vi "LogSummary.vi"(8 "error in (no error)":errorcluster, 9 "Run Ratios":T1 {"LEC13/12" format="%_4e"; "DTfrac" format="%#_3g"; "DT" format="%#_3g"; "CountErr" format="%#_3g"; "d13C" format="%_4g"; "C13/12" format="%_4e"; "C14/12" format="%_4e"; "C14/13" format="%_3e"; "C12Cor" format="%_3e"; "C13" format="%_3e"; "C13H/L" format="%#_3g"}, 10 "Run Summary":T2 {"C12LE" format="%_3e"; "C13LE" format="%_3e"; "C1312" format="%_3e"; "C12" format="%_3e"; "C13L" format="%_3e"; "C13H" format="%_3e"}, 11 "Log File Path":path) -> (0 "error out":errorcluster)   [LabVIEW 2013]
uses:
  SummaryData.ctl
  RunRatios.ctl
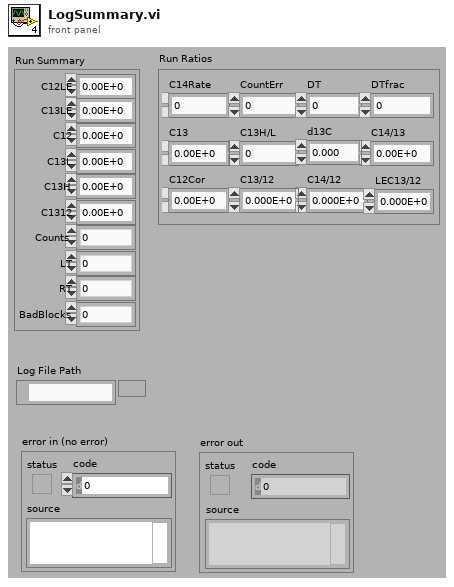
[diagram p1: front panel]
types:
  T1 = typedef "RunRatios.ctl" = cluster{"C14Rate":dbl, "CountErr":dbl, "DT":dbl, "DTfrac":dbl, "C13":dbl, "C13H/L":dbl, "d13C":dbl, "C14/13":dbl, "C12Cor":dbl, "C13/12":dbl, "C14/12":dbl, "LEC13/12":dbl}
  T2 = typedef "SummaryData.ctl" = cluster{"C12LE":dbl, "C13LE":dbl, "C12":dbl, "C13L":dbl, "C13H":dbl, "C1312":dbl, "Counts":u32, "LT":dbl, "RT":dbl, "BadBlocks":u8}
  T3 = enum16{"open", "replace", "create", "open or create", "replace or create", "replace or create with confirmation"}
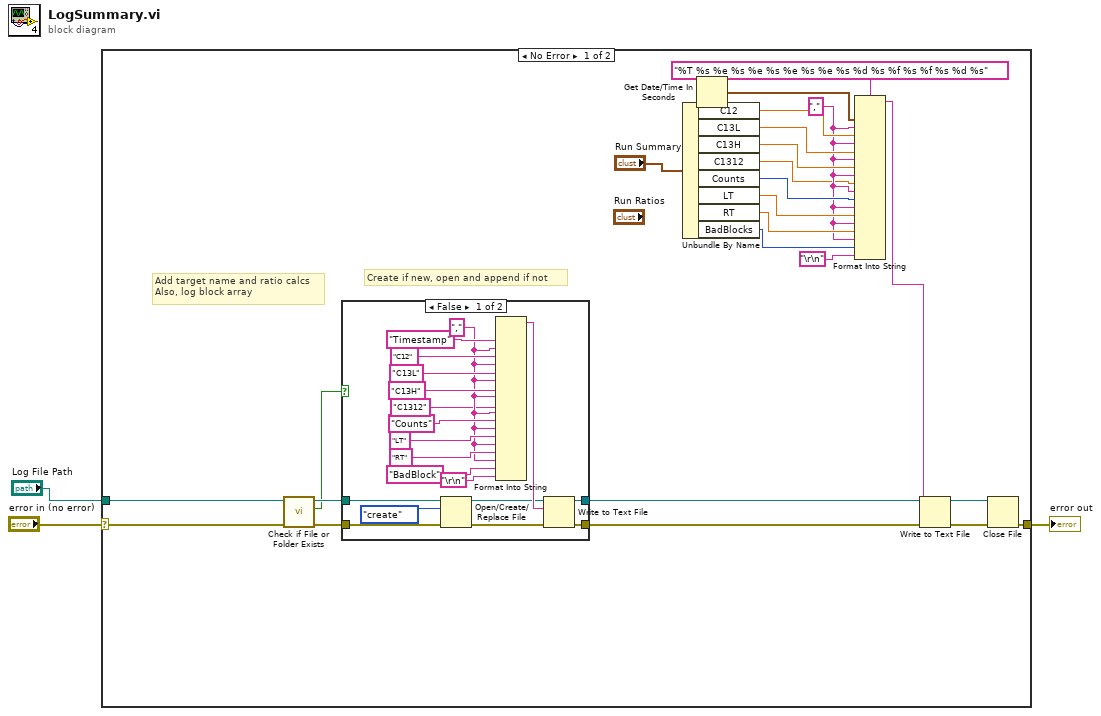
[diagram p0: block diagram]
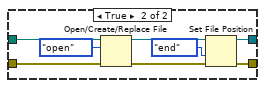
[diagram p2: hidden frame]
diagram:
  n1 = case shown="No Error" "error in (no error)" {
    selector: "error in (no error)" -> [w8 w55]
    tunnel: [w9 w55] -> w2
    tunnel: "Log File Path" -> [w4 _]
    frame No Error {
      w7 = ","
      # "Add target name and ratio calcs\nAlso, log block array"
      # "Create if new, open and append if not"
      n2 = call <vilib>:"Check if File or Folder Exists.vi"("error in (no error)"=w8, "path"=w4) -> ("error out"=w12:errorcluster, "file or folder exists?"=w10:bool, "dup path"=w13:path)  [unwired: 7 out]
      n3 = case shown="False" w10 {
        tunnel: [w33 w52] -> w16
        tunnel: [w32 w53] -> w11
        tunnel: w13 -> [w31 w49]
        tunnel: w12 -> [w30 w50]
        frame False {
          w29 = ","
          n4 = Open/Create/Replace File(file path (use dialog)=w31, error in=w30, operation (0:open)=T3."create") -> (refnum out=w35:refnum<file>, error out=w36:errorcluster)  [unwired: 4 out]
          n5 = Format Into String("Timestamp" ("input 1"), w29, "C12", w29, "C13L", w29, "C13H", w29, "C1312", w29, "Counts", w29, "LT", w29, "RT", w29, "BadBlock", "\r\n") -> (resulting string=w37:string)  [unwired: 3 in, 1 out]
          n6 = Write to Text File(file (use dialog)=w35, text=w37, error in=w36) -> (refnum out=w32:refnum<file>, error out=w33:errorcluster)  [unwired: 2 out]
        }
        frame True {
          n7 = Open/Create/Replace File(file path (use dialog)=w49, error in=w50, operation (0:open)=T3."open") -> (refnum out=w48:refnum<file>, error out=w51:errorcluster)  [unwired: 4 out]
          n8 = Set File Position(refnum=w48, from (0:start)=enum16{"start", "end", "current"}."end", error in=w51) -> (refnum out=w53:refnum<file>, error out=w52:errorcluster)  [unwired: 1 out]
        }
      }
      n9 = Unbundle By Name("Run Summary") -> ("C12"=w25:dbl, "C13L"=w24:dbl, "C13H"=w22:dbl, "C1312"=w6:dbl, "Counts"=w18:u32, "LT"=w19:dbl, "RT"=w20:dbl, "BadBlocks"=w21:u8)
      n10 = Get Date/Time In Seconds() -> (seconds since 1Jan1904=w23:timestamp)
      n11 = Format Into String(format string="%T %s %e %s %e %s %e %s %e %s %d %s %f %s %f %s %d %s", w23, w7, w25, w7, w24, w7, w22, w7, w6, w7, w18, w7, w19, w7, w20, w7, w21, "\r\n") -> (resulting string=w17:string)  [unwired: 2 in, 1 out]
      n12 = Write to Text File(file (use dialog)=w11, text=w17, error in=w16) -> (refnum out=w14:refnum<file>, error out=w15:errorcluster)  [unwired: 2 out]
      n13 = Close File(refnum=w14, error in=w15) -> (error out=w9:errorcluster)  [unwired: 1 out]
    }
    frame Error {
    }
  }
  "error out" <- w2
